vi "Kcotoo.vi"(11 "C":dbl) -> (3 "Numeric":dbl)   [LabVIEW 2022 SP3]
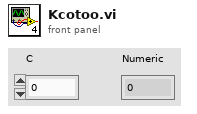
[diagram p1: front panel]
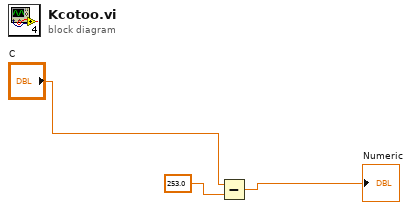
[diagram p0: block diagram]
diagram:
  n1 = Subtract(x="C", y=253.0) -> (x-y=→"Numeric":dbl)
